vi "Alarm Spike Delay.vi"(8 "Alarm Spike Delay (s)":dbl=10.0 format="%#_13g", 9 "Numeric Alarm Settings In":T1, 10 "Alarm Time In":cluster{"Name":string, "Alarm Time":timestamp}, 11 "Value In":dbl) -> (2 "Cluster out":cluster{"Name":string, "Alarm Time":timestamp}, 3 "Value Out":dbl)   [LabVIEW 2018, in "DAQ.lvlib"]
uses:
  DAQ.lvlib
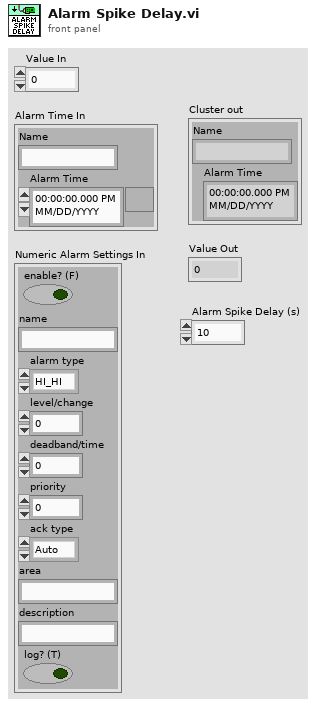
[diagram p1: front panel]
types:
  T1 = cluster{"enable? (F)":bool, "name":string, "alarm type":enum16{"HI_HI", "HI", "LO", "LO_LO"}, "level/change":dbl, "deadband/time":dbl, "priority":u32, "ack type":enum16{"Auto", "User", "None", "Each Occurrence"}, "area":string, "description":string, "log? (T)":bool}
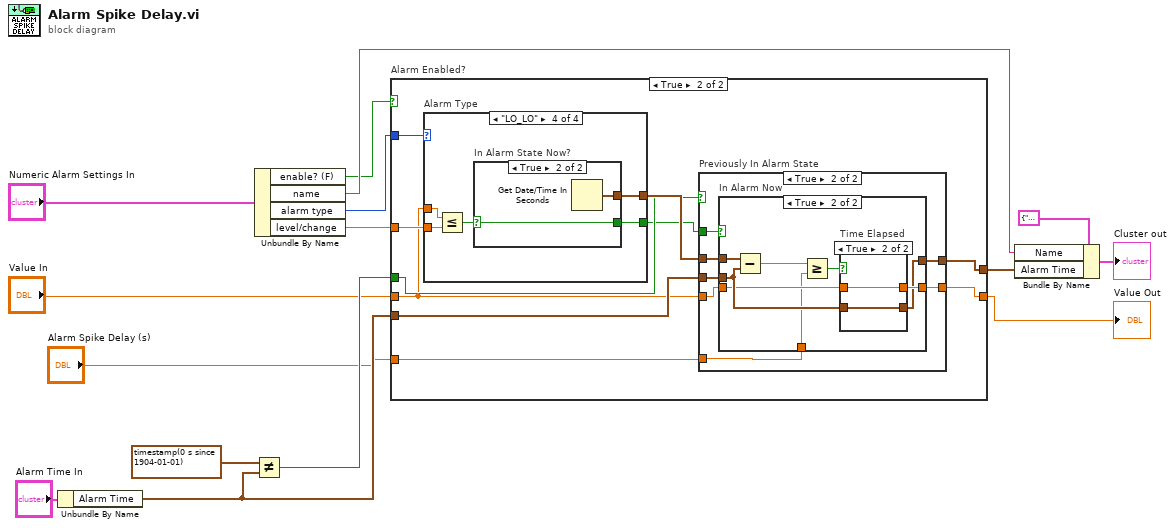
[diagram p0: block diagram]
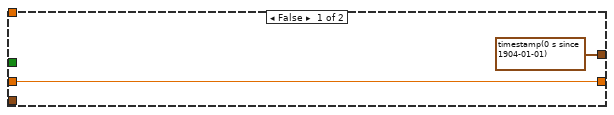
[diagram p2: hidden frame]
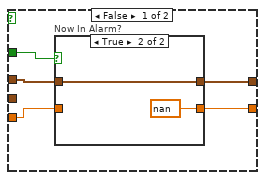
[diagram p3: hidden frame]
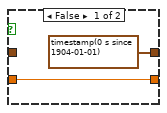
[diagram p4: hidden frame]
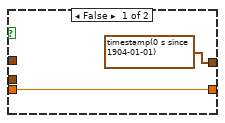
[diagram p5: hidden frame]
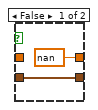
[diagram p6: hidden frame]
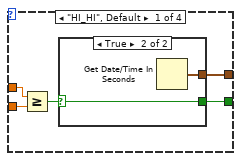
[diagram p7: hidden frame]
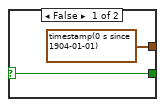
[diagram p8: hidden frame]
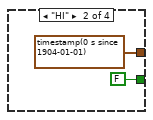
[diagram p9: hidden frame]
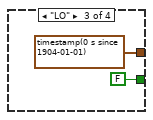
[diagram p10: hidden frame]
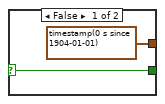
[diagram p11: hidden frame]
diagram:
  n1 = Unbundle By Name("Alarm Time In") -> ("Alarm Time"=w14:timestamp)
  n2 = Not Equal?(x=timestamp(0 s since 1904-01-01), y=w14) -> (x != y?=w13:bool)
  n3 = Unbundle By Name("Numeric Alarm Settings In") -> ("enable? (F)"=w3:bool, "name"=w9:string, "alarm type"=w4:enum16{"HI_HI", "HI", "LO", "LO_LO"}, "level/change"=w5:dbl)
  n4 = case "Alarm Enabled?" shown="True" w3 {
    tunnel: w4 -> [_ w27]
    tunnel: w5 -> [_ w26]
    tunnel: "Value In" -> [w16 w19]
    tunnel: [timestamp(0 s since 1904-01-01) w22] -> w12
    tunnel: w13 -> [_ w24]
    tunnel: w14 -> [_ w23]
    tunnel: [w16 w20] -> w15
    tunnel: "Alarm Spike Delay (s)" -> [_ w18]
    frame False {
    }
    frame True {
      n5 = case "Alarm Type" shown="\"LO_LO\"" w27 {
        tunnel: w26 -> [w62 _ _ w72]
        tunnel: w19 -> [w61 _ _ w73]
        tunnel: [w60 timestamp(0 s since 1904-01-01) ("seconds since 1Jan1904") timestamp(0 s since 1904-01-01) ("seconds since 1Jan1904") w74] -> w25
        tunnel: [w58 FALSE FALSE w71] -> w21
        frame "HI_HI", Default {
          n6 = Greater Or Equal?(x=w61, y=w62) -> (x >= y?=w59:bool)
          n7 = case shown="True" w59 {
            selector: w59 -> [w63 w65]
            tunnel: [timestamp(0 s since 1904-01-01) ("seconds since 1Jan1904") w66] -> w60
            tunnel: [w63 w65] -> w58
            frame False {
            }
            frame True {
              n8 = Get Date/Time In Seconds() -> (seconds since 1Jan1904=w66:timestamp)
            }
          }
        }
        frame "HI" {
        }
        frame "LO" {
        }
        frame "LO_LO" {
          n9 = Less Or Equal?(x=w73, y=w72) -> (x <= y?=w75:bool)
          n10 = case "In Alarm State Now?" shown="True" w75 {
            selector: w75 -> [w76 w78]
            tunnel: [timestamp(0 s since 1904-01-01) ("seconds since 1Jan1904") w79] -> w74
            tunnel: [w76 w78] -> w71
            frame False {
            }
            frame True {
              n11 = Get Date/Time In Seconds() -> (seconds since 1Jan1904=w79:timestamp)
            }
          }
        }
      }
      n12 = case "Previously In Alarm State" shown="True" w24 {
        tunnel: w25 -> [w30 w43]
        tunnel: w23 -> [_ w42]
        tunnel: [w31 w38] -> w22
        tunnel: w21 -> [w32 w41]
        tunnel: [w29 w39] -> w20
        tunnel: w19 -> [w28 w40]
        tunnel: w18 -> [_ w37]
        frame False {
          n13 = case "Now In Alarm?" shown="True" w32 {
            tunnel: [timestamp(0 s since 1904-01-01) ("seconds since 1Jan1904") w36] -> w31
            tunnel: w30 -> [_ w36]
            tunnel: [w34 nan] -> w29
            tunnel: w28 -> [w34 _]
            frame False {
            }
            frame True {
            }
          }
        }
        frame True {
          n14 = case "In Alarm Now" shown="True" w41 {
            tunnel: w43 -> [_ w53]
            tunnel: w42 -> [_ w49]
            tunnel: w40 -> [w45 w47]
            tunnel: [w45 w50] -> w39
            tunnel: [timestamp(0 s since 1904-01-01) ("seconds since 1Jan1904") w48] -> w38
            tunnel: w37 -> [_ w46]
            frame False {
            }
            frame True {
              n15 = Subtract(x=w53, y=w49) -> (x-y=w51:dbl)
              n16 = Greater Or Equal?(x=w51, y=w46) -> (x >= y?=w52:bool)
              n17 = case "Time Elapsed" shown="True" w52 {
                tunnel: [nan w57] -> w50
                tunnel: w49 -> [w54 w56]
                tunnel: [w54 w56] -> w48
                tunnel: w47 -> [_ w57]
                frame False {
                }
                frame True {
                }
              }
            }
          }
        }
      }
    }
  }
  "Value Out" <- w15
  n18 = Bundle By Name(cluster=cluster{"Name":string, "Alarm Time":timestamp} {"Name"="", "Alarm Time"=timestamp(0 s since 1904-01-01)}, "Name"=w9, "Alarm Time"=w12) -> (→"Cluster out":cluster{"Name":string, "Alarm Time":timestamp})
